vi "Add Overflow Support FXP(+-,14,1)x4ch.vi"(3 "overflow":bool, 4 "data in":T1={"channel 0"=[0.0, 0.0], "channel 1"=[0.0, 0.0], "channel 2"=[0.0, 0.0], "channel 3"=[0.0, 0.0]}) -> (1 "data out":T1)   [LabVIEW 2014]
doc: "Adds overflow to input data.\n\n<B>Supported data types</B>\nFXP +-,18,1; FXP +-,14,1\n\n<B>Supported channel size</B>\n4, 8\n\n<B>Supported samples per cycle</B>\n2\n\n<B>Input Parameters</B>\n\n<B>data in</B> specifies the data input without the overflow.\n\n<B>overflow</B> specifies the overflow to add to the input data.\n\n<B>Output Parameters</B>\n\n<B>data out</B> returns the data with overflow added."
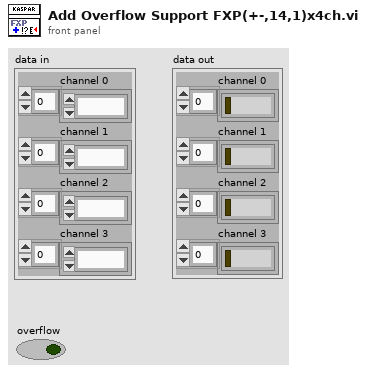
[diagram p1: front panel]
types:
  T1 = cluster{"channel 0":fxp<+/-,14,1>[], "channel 1":fxp<+/-,14,1>[], "channel 2":fxp<+/-,14,1>[], "channel 3":fxp<+/-,14,1>[]}
  T2 = cluster{"data out":fxp<+/-,14,1>[], "data out":fxp<+/-,14,1>[], "data out":fxp<+/-,14,1>[], "data out":fxp<+/-,14,1>[]}
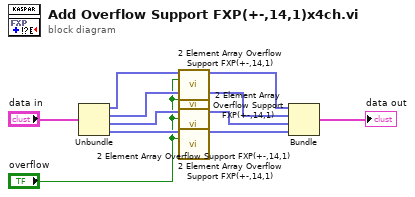
[diagram p0: block diagram]
diagram:
  n1 = Unbundle("data in") -> ("channel 0"=w6:fxp<+/-,14,1>[], "channel 1"=w5:fxp<+/-,14,1>[], "channel 2"=w4:fxp<+/-,14,1>[], "channel 3"=w3:fxp<+/-,14,1>[])
  n2 = call "2 Element Array Overflow Support FXP(+-,14,1).vi"("data in"=w6, "overflow"="overflow") -> ("data out"=w11:fxp<+/-,14,1>[])  [unwired: 13 in]
  n3 = call "2 Element Array Overflow Support FXP(+-,14,1).vi"("data in"=w5, "overflow"="overflow") -> ("data out"=w10:fxp<+/-,14,1>[])  [unwired: 13 in]
  n4 = call "2 Element Array Overflow Support FXP(+-,14,1).vi"("data in"=w4, "overflow"="overflow") -> ("data out"=w9:fxp<+/-,14,1>[])  [unwired: 13 in]
  n5 = call "2 Element Array Overflow Support FXP(+-,14,1).vi"("data in"=w3, "overflow"="overflow") -> ("data out"=w8:fxp<+/-,14,1>[])  [unwired: 13 in]
  n6 = Bundle("data out"=w11, "data out"=w10, "data out"=w9, "data out"=w8) -> (→"data out":T2)  [unwired: 1 in]
